vi "Mysql command.vi"(8 "error in (no error)":errorcluster, 10 "Query string":string, 11 "mysql in":refnum<class "mysql.lvclass">) -> (0 "error out":errorcluster, 3 "ExecuteReader":refnum<k24>)   [LabVIEW 2020, in "mysql.lvlib" / "mysql.lvclass"]
uses:
  mysql.lvclass
  MySql.Data
  mysql.lvclass/mysql.ctl
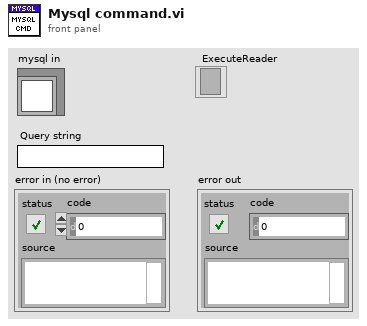
[diagram p1: front panel]
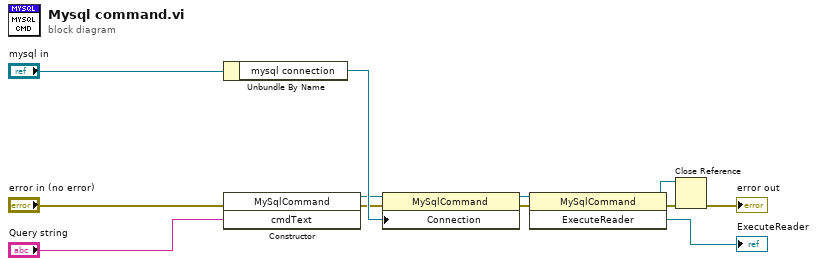
[diagram p0: block diagram]
diagram:
  n1 = Unbundle By Name("mysql in") -> ("mysql connection"=w11:refnum<k24>)
  n2 = constructor class="MySqlCommand"(error in="error in (no error)", "cmdText"="Query string") -> (reference out=w8:refnum<k24>, error out=w7:errorcluster)  [unwired: 2 in, 2 out]
  n3 = property class="MySqlCommand"(reference=w8, error in=w7, "Connection"=w11) -> (reference out=w9:refnum<k24>, error out=w6:errorcluster)
  n4 = invoke class="MySqlCommand" method="ExecuteReader"(reference=w9, error in=w6) -> (reference out=w2:refnum<k24>, error out=w12:errorcluster, "ExecuteReader"=→"ExecuteReader":refnum<k24>)  [unwired: 1 in]
  n5 = Close Reference(reference=w2, error in (no error)=w12) -> (error out=→"error out":errorcluster)
